vi "Get Product.vi"(8 "error in (no error)":errorcluster, 10 "Producto":string, 11 "User Interface in":refnum<class "User Interface.lvclass">) -> (0 "error out":errorcluster, 3 "User Interface out":refnum<class "User Interface.lvclass">)   [LabVIEW 2020, in "User Interface.lvlib" / "User Interface.lvclass"]
uses:
  User Interface.lvclass
  Manejador de Turnos Messages/Set the Turn Msg/Set the Turn Msg.lvclass
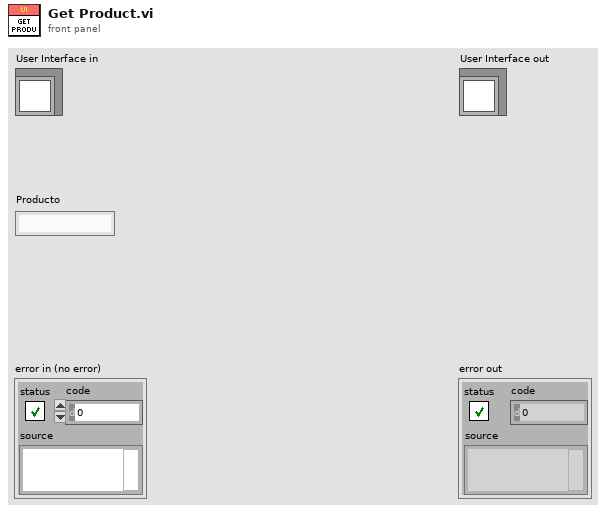
[diagram p1: front panel]
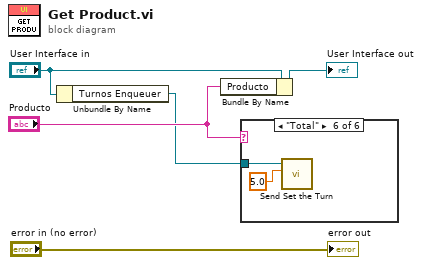
[diagram p0: block diagram]
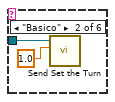
[diagram p3: hidden frame]
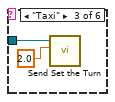
[diagram p4: hidden frame]
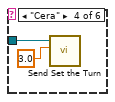
[diagram p5: hidden frame]
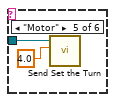
[diagram p6: hidden frame]
diagram:
  n1 = Unbundle By Name("User Interface in") -> ("Turnos Enqueuer"=w1:refnum<class "Message Enqueuer.lvclass">)
  n2 = Bundle By Name(cluster="User Interface in", "Producto"="Producto") -> (→"User Interface out":refnum<class "User Interface.lvclass">)
  n3 = case shown="\"Total\"" "Producto" {
    tunnel: w1 -> [_ w7 w9 w11 w13 w15]
    frame " ", Default {
    }
    frame "Basico" {
      n4 = call "Send Set the Turn.vi"("Selector"=1.0, "Message Enqueuer"=w7) -> ()  [unwired: 8 in, 2 out]
    }
    frame "Taxi" {
      n5 = call "Send Set the Turn.vi"("Selector"=2.0, "Message Enqueuer"=w9) -> ()  [unwired: 8 in, 2 out]
    }
    frame "Cera" {
      n6 = call "Send Set the Turn.vi"("Selector"=3.0, "Message Enqueuer"=w11) -> ()  [unwired: 8 in, 2 out]
    }
    frame "Motor" {
      n7 = call "Send Set the Turn.vi"("Selector"=4.0, "Message Enqueuer"=w13) -> ()  [unwired: 8 in, 2 out]
    }
    frame "Total" {
      n8 = call "Send Set the Turn.vi"("Selector"=5.0, "Message Enqueuer"=w15) -> ()  [unwired: 8 in, 2 out]
    }
  }
  "error out" <- "error in (no error)"
